vi "Read XML_Extra Checks_Check Parameter Parity Bit Tx.vi"(8 "error in (no error)":errorcluster, 11 "Channels In":T1[](array[typedef])) -> (0 "error out":errorcluster)   [LabVIEW 2017]
doc: "This VI checks that no Tx Labels have Parity Bit exposed. It's not allowed. In case there are occurences, there is a 5014 error returned."
uses:
  XML_Channel.ctl
  XML_Label.ctl
  XML_Parameter.ctl
  <userlib>/_OpenG.lib/array/array.llb/Filter 1D Array with Scalar (Boolean)__ogtk.vi
panel:
  out "Error Source":string
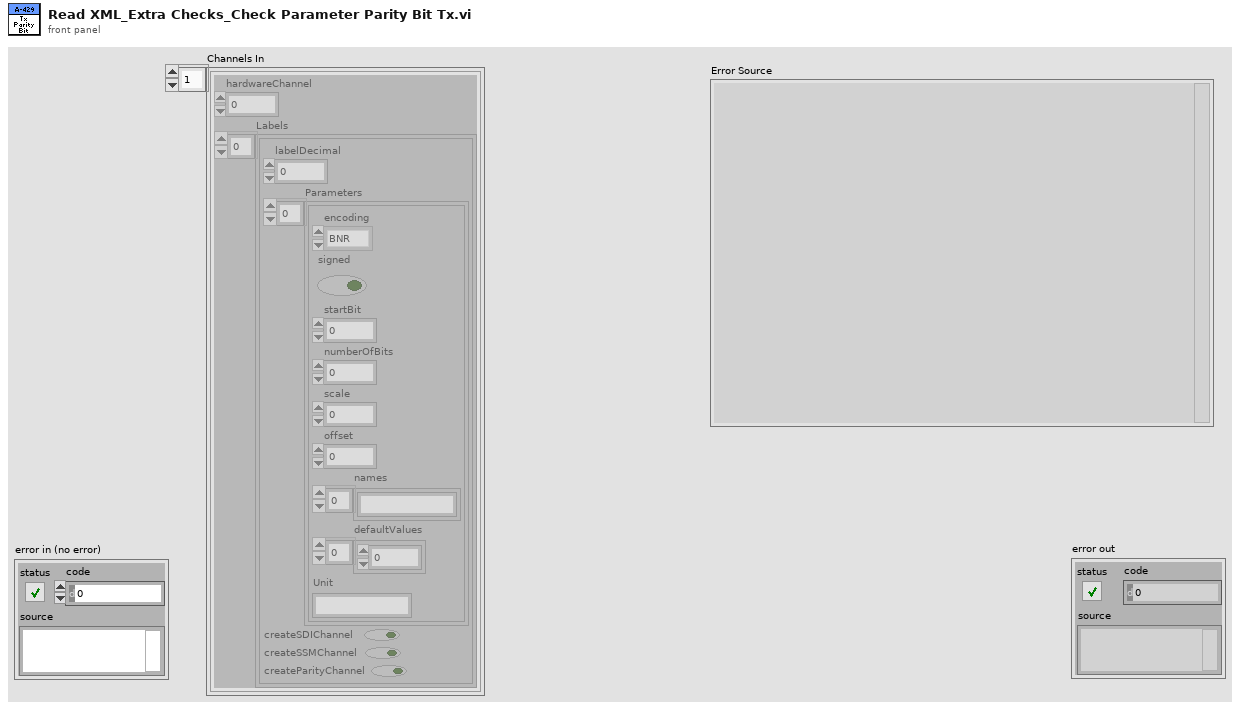
[diagram p1: front panel]
types:
  T1 = typedef "XML_Channel.ctl" = cluster{"hardwareChannel":i32, "Labels":T2[]}
  T2 = typedef "XML_Label.ctl" = cluster{"labelDecimal":i32, "Parameters":T3[], "createSDIChannel":bool, "createSSMChannel":bool, "createParityChannel":bool}
  T3 = typedef "XML_Parameter.ctl" = cluster{"encoding":enum16{"BNR", "BCD", "Discrete"}, "signed":bool, "startBit":i32, "numberOfBits":i32, "scale":dbl, "offset":dbl, "names":string[], "defaultValues":dbl[], "Unit":string}
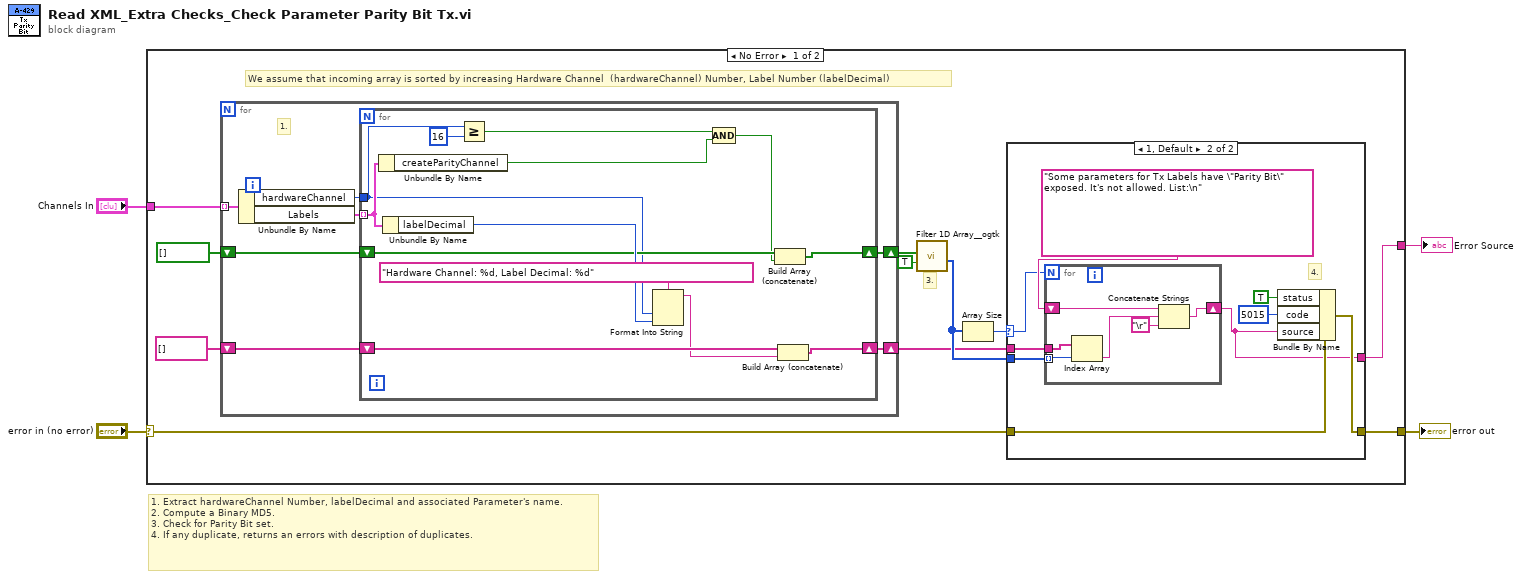
[diagram p0: block diagram]
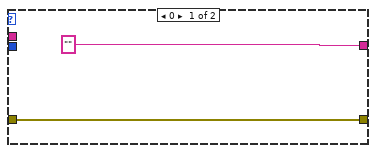
[diagram p2: hidden frame]
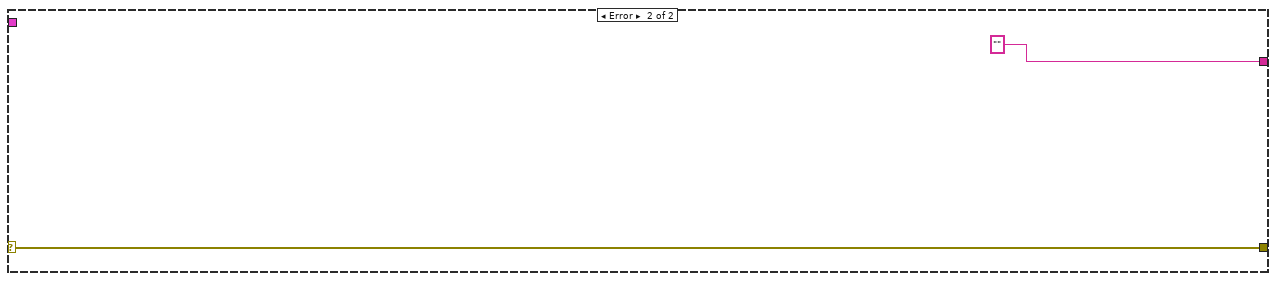
[diagram p3: hidden frame]
diagram:
  # "1. Extract hardwareChannel Number, labelDecimal and associated Parameter's name.\n2. Compute a Binary MD5.\n3. Check for Parity Bit set.\n4. If any duplicate, returns an errors with description of duplicates."
  n1 = case shown="No Error" "error in (no error)" {
    selector: "error in (no error)" -> [w14 w54]
    tunnel: [w11 w54] -> w3
    tunnel: "Channels In" -> [w13 _]
    tunnel: [w10 ""] -> w1
    frame No Error {
      # "3."
      # "We assume that incoming array is sorted by increasing Hardware Channel  (hardwareChannel) Number, Label Number (labelDecimal)"
      n2 = for {
        tunnel: w13 -> [w39] mode=indexing
        shift-right: [w35] -> w7
        shift-left: bool[] [] -> [w36]
        shift-right: [w33] -> w8
        shift-left: string[] [] -> [w34]
        # "1."
        n3 = Unbundle By Name(w39) -> ("hardwareChannel"=w38:i32, "Labels"=w37:T2[])
        n4 = for {
          tunnel: w38 -> [w45]
          tunnel: w37 -> [w47] mode=indexing
          shift-right: [w50] -> w35
          shift-left: w36 -> [w51]
          shift-right: [w48] -> w33
          shift-left: w34 -> [w49]
          n5 = Unbundle By Name(w47) -> ("createParityChannel"=w46:bool)
          n6 = Unbundle By Name(w47) -> ("labelDecimal"=w52:i32)
          n7 = Greater Or Equal?(x=w45, y=16) -> (x >= y?=w43:bool)
          n8 = Format Into String(format string="Hardware Channel: %d, Label Decimal: %d", w45, w52) -> (resulting string=w41:string)  [unwired: 2 in, 1 out]
          n9 = Compound Arithmetic op=AND(w43, w46) -> (w40:bool)
          n10 = Build Array (concatenate)(w51, w40) -> (w50:bool[])
          n11 = Build Array (concatenate)(w49, w41) -> (w48:string[])
        }
      }
      n12 = call-poly <userlib>:"Filter 1D Array__ogtk.vi"("items to filter"=TRUE, "array"=w7) -> ("filtered item indices"=w12:i32[])  [unwired: 4 in, 1 out]
      n13 = Array Size(array=w12) -> (size(s)=w15:i32)
      n14 = case shown="1, Default" w15 {
        selector: w15 -> [_ w21]
        tunnel: w14 -> [w17 w26]
        tunnel: w12 -> [_ w20]
        tunnel: [w17 w25] -> w11
        tunnel: ["" w19] -> w10
        tunnel: w8 -> [_ w18]
        frame 0 {
        }
        frame 1, Default {
          # "4."
          n15 = for {
            N: w21 -> [_]
            shift-right: [w31] -> w19
            shift-left: "Some parameters for Tx Labels have \"Parity Bit\" exposed. It's not allowed. List:\n" -> [w32]
            tunnel: w20 -> [w30] mode=indexing
            tunnel: w18 -> [w28]
            n16 = Index Array(array=w28, index=w30) -> (element=w27:string)
            n17 = Concatenate Strings(w32, w27, "\r") -> (w31:string)
          }
          n18 = Bundle By Name(cluster=w26, "status"=TRUE, "code"=5015, "source"=w19) -> (w25:errorcluster)
        }
      }
    }
    frame Error {
    }
  }
  "error out" <- w3
  "Error Source" <- w1
